vi "Peak Detector.vi"   [LabVIEW 2016, in "xy_utilities.lvlib"]
doc: "Find <b>peaks</b> in <b>XY-data</b>'s Y-Array.\n\nWire data to the data input to determine the polymorphic instance to use or manually select the instance."
uses:
  xy_utilities.lvlib
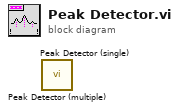
[diagram p0: block diagram]
diagram:
  n1 = call "Peak Detector (multiple).vi"() -> ()  [unwired: 8 in, 4 out]
  n2 = call "Peak Detector (single).vi"() -> ()  [unwired: 8 in, 4 out]
